vi "Read Request.vi"(8 "error in (no error)":errorcluster, 9 "Request File Name":string) -> (0 "error out":errorcluster, 1 "Good Method":bool, 2 "User and project info":T2, 3 "Byte Stream File out":refnum<file>, 5 "Method Name":string)   [LabVIEW 2011, in "Design Server.lvlib"]
uses:
  Design Server.lvlib
  user project design.ctl
  Variable cluster.ctl
  Folders.ctl
panel:
  out "data":T1
  in  "request datatype":T1
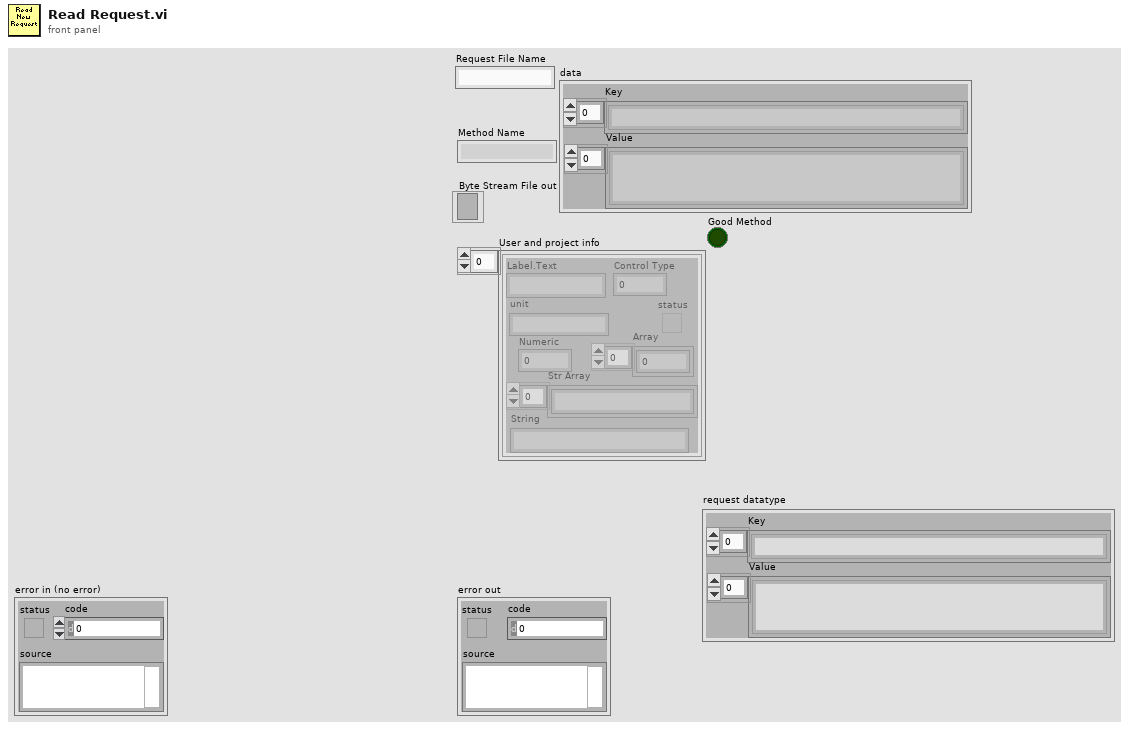
[diagram p1: front panel]
types:
  T1 = typedef "Design Server.lvlib/user project design.ctl" = cluster{"Key":string[], "Value":string[]}
  T2 = typedef "Design Server.lvlib/Variable cluster.ctl" = cluster{"Label.Text":string, "Control Type":u32, "Numeric":dbl, "Array":dbl[], "status":bool, "Str Array":string[], "String":string, "unit":string}[]
  T3 = typedef "Design Server.lvlib/Folders.ctl" = enum16{"MathcadMethods", "RequestedDesigns", "CompletedDesigns", "MathcadCode", "CollabnetSVN.exe"}
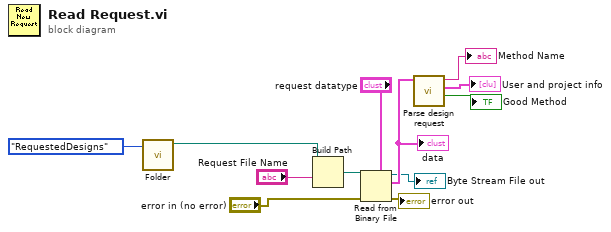
[diagram p0: block diagram]
diagram:
  n1 = call "Folder.vi"("Folders"=Folders."RequestedDesigns") -> ("FolderPath"=w2:path)  [unwired: 8 in, 2 out]
  n2 = Build Path(base path=w2, name or relative path="Request File Name") -> (appended path=w5:path)
  n3 = Read from Binary File(5:"request datatype", 8:"error in (no error)", 11:w5) -> (0:→"error out":errorcluster, 2:w8:T1, 3:→"Byte Stream File out":refnum<file>)  [unwired: 3 in, 1 out]
  "data" <- w8
  n4 = call "Parse design request.vi"("Request"=w8) -> ("Good Method"=→"Good Method":bool, "User and project info"=→"User and project info":T2, "Method"=→"Method Name":string)  [unwired: 8 in]
